vi "SubVI_CaptureVIS.vi"(0 "ErrorIn":errorcluster, 5 "au8Channel-B":u8[](array[numeric]), 9 "au8Channel-G":u8[](array[numeric]), 11 "au8Channel-R":u8[](array[numeric])) -> (1 "i32VisHeight":i32, 3 "i32VisWidth":i32, 4 "ErrorOut":errorcluster, 6 "au8Channel-B":u8[](array[numeric]), 10 "au8Channel-G":u8[](array[numeric]), 14 "u8Error":u8, 15 "au8Channel-R":u8[](array[numeric]))   [LabVIEW 2013]
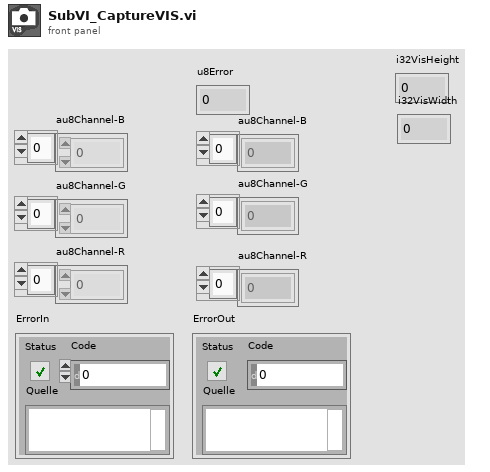
[diagram p1: front panel]
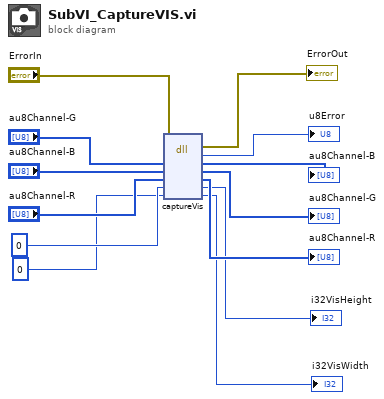
[diagram p0: block diagram]
diagram:
  n1 = dll-call lib="PTH1abs CUsers1000len-bimDesktop&Lieferung_LabView_Interface_11.11.2015Einrichten fÃ¼r - EndkundenDatenTesto_v2013VIlabview_cwrapper_1_0_0.dll" fn="captureVis"(error in="ErrorIn", "au8ChannelB"="au8Channel-G", "au8ChannelG"="au8Channel-B", "au8ChannelR"="au8Channel-R", "i32VisHeight"=0 ("i32VisWidth"), "i32VisWidth"=0) -> (error out=→"ErrorOut":errorcluster, "u8Error"=→"u8Error":u8, "au8ChannelB"=→"au8Channel-B":u8[], "au8ChannelG"=→"au8Channel-G":u8[], "au8ChannelR"=→"au8Channel-R":u8[], "i32VisHeight"=→"i32VisHeight":i32, "i32VisWidth"=→"i32VisWidth":i32)  [unwired: 2 in, 1 out]
